vi "Friendly Name.vi"(8 "error in (no error)":errorcluster, 11 "VisaResource in":refnum<class "VisaResource.lvclass">) -> (0 "error out":errorcluster, 2 "Friendly Name":string, 3 "VisaResource out":refnum<class "VisaResource.lvclass">)   [LabVIEW 2020, in "VisaResource.lvclass"]
uses:
  VisaResource.lvclass
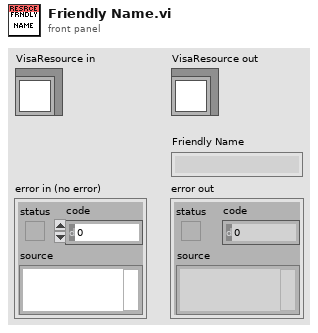
[diagram p1: front panel]
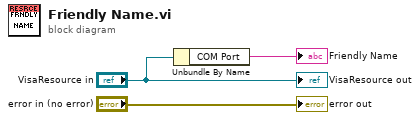
[diagram p0: block diagram]
diagram:
  n1 = Unbundle By Name("VisaResource in") -> ("COM Port"=→"Friendly Name":string)
  "error out" <- "error in (no error)"
  "VisaResource out" <- "VisaResource in"
